vi "E517_Wavegen_Example.vi"(0 "System no.":i32=1 min=1 step=1, 1 "# Wavegenerators":i32, 2 "Programmatic events":T1(array[ring]), 5 "error in":errorcluster, 6 "Enabled":bool[](array[boolean])=[FALSE, FALSE, FALSE, FALSE, FALSE, FALSE, FALSE, FALSE], 7 "# WG cycles":i32[](array[numeric]) format="%#.0f", 9 "SIN_P parameters":cluster{"C":dbl, "A":dbl, "O":dbl}={"C"=500.0, "A"=5.0, "O"=0.0} {"O" format="%.6f"; "A" format="%.6f"; "C" format="%.6f"}, 11 "Firing Wavepoints":i32[][](array[numeric])=[[100, 550], [200, 450], [300, 350]] format="%#.0f", 13 "Append?":bool) -> (16 "Triggerpoints":dbl[][](graph), 17 "Wavetable data":dbl[][](graph), 18 "Recordtable data":dbl[][](graph), 19 "Error out":errorcluster)   [LabVIEW 2011]
doc: "This VI demonstrates how to configure the wave generator, set wave tables, read data recorder tables and set trigger points. The diagram shows how to combine the driver VIs for these tasks. \nThe controls connected to the connector pane exemplify the application. You can modify the connector pane and add controls to meet your requirements. The E517_Wavegen_Example_Caller.vi shows how to call this VI programmatically as a SubVI.\n\nRun E517_Configuration_Setup.vi prior to running this VI.\n\nOn the [Settings] tab you can link wave tables to wave generators if this feature is supported by your controller, adjust wave table and record table rates and configure the wave generator. The current wave generator mode setting (WGO), the actual positions and the servo states are updated continuously.\n \nSelect the desired wave table on the [Wavetables] tab to write a waveform into it or to clean a previously stored waveform. #points in WT shows the actual length of the tables. You can apply controller generated sine waves or host PC generated point-by-point ramp waveforms covering the motion range of the appropriate connected stage. Please consult the Context Help window of the WAV.vi the User Manual of your controller for details on waveform settings. After writing a waveform to the controller all waveforms are read back and displayed automatically. You can read out the wave tables manually, too.\n\nAll further tabs are disabled until you have defined one wave table at least.\n \nConfigure the data recorder on the [Recordtables] tab prior to reading out any data. Each data recorder table must be configured separately by choosing a linked axis and an axis related record option. The contents of the data recorder tables are not read out automatically. Reasonable data is only available if at least one wave generator run has been started since the last power-on / reboot of the controller.\n \nOn the [Triggerpoints] tab you can link axes to triggerlines if this feature is supported by your controller. If you want to output trigger pulses synchronized with the wave generator output, activate the Generator Trigger mode by pressing the Set TWS trigger mode button. The trigger related controls will then be activated. In the matrix you can define the active trigger points for each triggerline. They will be written to the controller's RAM by Set these trigger points. To reset trigger points use Clear all trigger points. In the graphics pane the active trigger points are displayed as bars."
panel:
  out "Number of Triggerlines":i32
  out "SubVI":bool
  out "Running?":bool[](array[boolean])
  in  "Tab Control":T2(tab)
  out "Axes":string[](array[string])
  in  "Recordtable rate":i32=1
  in  "Wavegen":i32[](array[numeric])=[1, 2, 3] format="%#.0f"
  out "# Recordtables":i32
  out "# Wavetables":i32
  out "# Wavegenerators":i32
  out "Servo":bool[](array[boolean])
  in  "Wavetable rate":i32[](array[numeric]) format="%#.0f"
  out "Positions":dbl[](array[numeric])
  out "WGO mode":i32[](array[numeric]) format="%#.0f"
  in  "Start at\nEndpoint":bool[](array[boolean])=[FALSE, FALSE, FALSE, FALSE, FALSE, FALSE, FALSE, FALSE]
  in  "DDL init":bool[](array[boolean])=[FALSE, FALSE, FALSE, FALSE, FALSE, FALSE, FALSE, FALSE]
  in  "DDL enable":bool[](array[boolean])=[FALSE, FALSE, FALSE, FALSE, FALSE, FALSE, FALSE, FALSE]
  in  "Segm.Length":i32=1000
  in  "GWD?":bool
  out "# points in WT":i32[](array[numeric]) format="%#.0f"
  in  "WCL":bool
  out "PNT parameters (indicator)":cluster{"Ao..An-1":dbl[]}
  in  "Write sine":bool
  in  "Add?":bool
  in  "Xo":i32=1
  in  "N":i32=1000
  in  "Write points":bool
  out "Assigned\nwavegenerator":i32
  in  "Wavetable":u16(ring) items=["1", "2", "3"]
  in  "DRC?":bool
  out "Record option":string[](array[string])
  out "Source ID":string[](array[string])
  in  "DRC":bool
  in  "Record option":u16(ring)=1 items=["Target position of axis "=1, "Current position of axis "=2, "Position error of axis "=3, "Voltage of piezo channel "=7, "Control output of axis "=15]
  in  "Axis":u16(ring) items=["A", "B", "C"]
  in  "Record table":u16(ring) items=["1", "2", "3"]
  in  "N:":i32=1000
  in  "X0:":i32=1
  in  "DRR?":bool
  in  "CTO":bool
  in  "TWC":bool
  in  "TWS":bool
  in  "TWS?":bool
  in  "Axis":u16[](array[ring]) items=["A", "B", "C"]
  in  "Clear error":bool
  in  "Stop":bool
  # "E-517 wave generator, data recorder and trigger setting sample program"
  # "This VI demonstrates how to configure the wave generator, set wavetables, read recordtables and set triggerpoints.\nYou can apply controller generated sine waves or host PC generated point-by-point ramp waveforms.\nRun E517_Configuration_Setup.vi prior to running this VI."
  # "Wavegenerator state:"
  # "Wavetable"
  # "1"
  # "2"
  # "3"
  # "4"
  # "5"
  # "6"
  # "7"
  # "8"
  # "Wavegen"
  # "1"
  # "2"
  # "3"
  # "4"
  # "5"
  # "6"
  # "7"
  # "8"
  # "1"
  # "2"
  # "3"
  # "4"
  # "5"
  # "6"
  # "7"
  # "8"
  # "1black 2red 3green 4cyan 5yelllow 6purple 7orange 8blue"
  # "1"
  # "2"
  # "3"
  # "4"
  # "5"
  # "6"
  # "7"
  # "8"
  # "1black 2red 3green 4cyan 5yelllow 6purple 7orange 8blue"
  # "Trigger"
  # "1"
  # "2"
  # "3"
  # "4"
  # "5"
  # "6"
  # "1black 2red 3green 4blue 5yelllow 6purple"
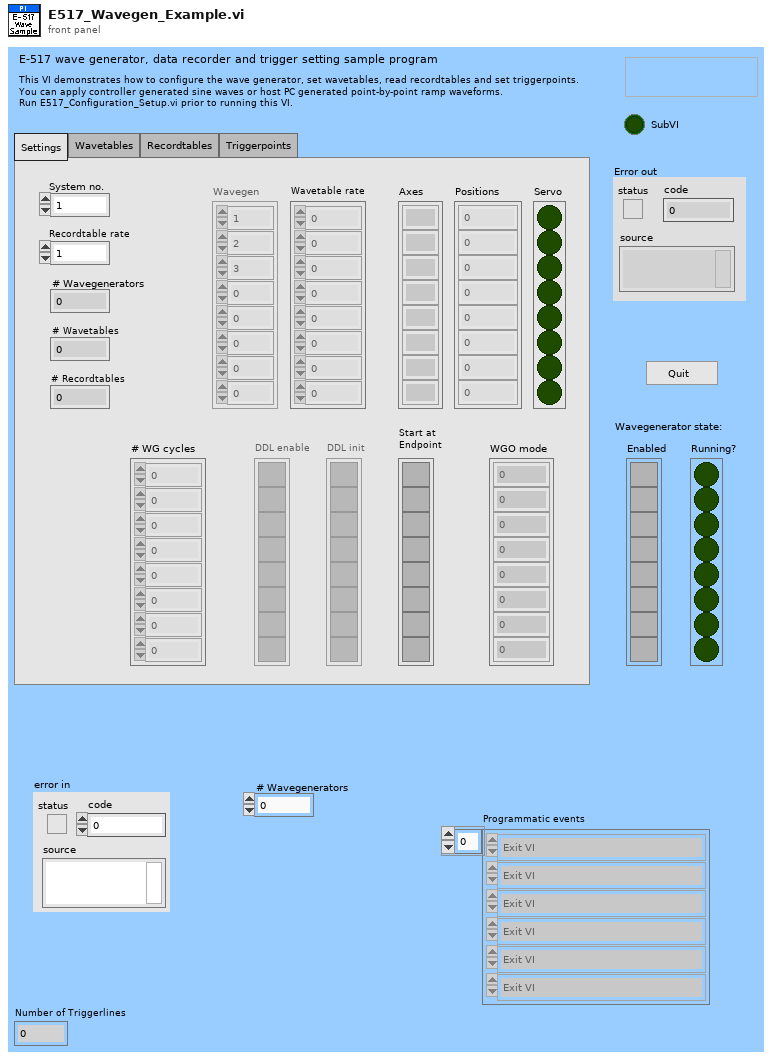
[diagram p1: front panel]
types:
  T1 = enum16{"Exit VI", "Set trigger mode", "Set recordtable rate", "Set wavetable rate", "Write sine", "Read wavetable", "Read recordtable", "Enable/disable wavegen", "Set number of wavegen cycles", "Clear wavetable", "Configure data recorder", "Assign wavetable to wavegen", "Read trigger points", "Set trigger points", "Clear trigger points", "Assign axes to triggerlines", "Write ramp waveform", "Set DDL enable", "Set DDL init", "Set Start at endpoint"}[]
  T2 = enum32{"Settings", "Wavetables", "Recordtables", "Triggerpoints"}
  T3 = enum32{"Page Enabled", "Page Disabled", "Page Disabled & Grayed"}
  T4 = enum16{"Position Distance", "Position Distance & Wait Time", "OnTarget", "MinMax Threshold", "Generator Trigger (TWS)", "Motion Error", "In Motion"}
  T5 = enum16{"Unused", "TriggerStep", "Axis", "TriggerMode", "TriggerDelay", "MinThreshold", "MaxThreshold", "Polarity", "StartThreshold", "StopThreshold"}
  T6 = enum16{"Position Distance", "Position Distance & Wait Time", "OnTarget", "MinMax Threshold", "Generator Trigger (TWS)", "Motion Error", "In Motion"}[]
  T7 = enum16{"Unused", "TriggerStep", "Axis", "TriggerMode", "TriggerDelay", "MinThreshold", "MaxThreshold", "Polarity", "StartThreshold", "StopThreshold"}[]
  T8 = enum16{"Exit VI", "Set trigger mode", "Set recordtable rate", "Set wavetable rate", "Write sine", "Read wavetable", "Read recordtable", "Enable/disable wavegen", "Set number of wavegen cycles", "Clear wavetable", "Configure data recorder", "Assign wavetable to wavegen", "Read trigger points", "Set trigger points", "Clear trigger points", "Assign axes to triggerlines", "Write ramp waveform", "Set DDL enable", "Set DDL init", "Set Start at endpoint"}
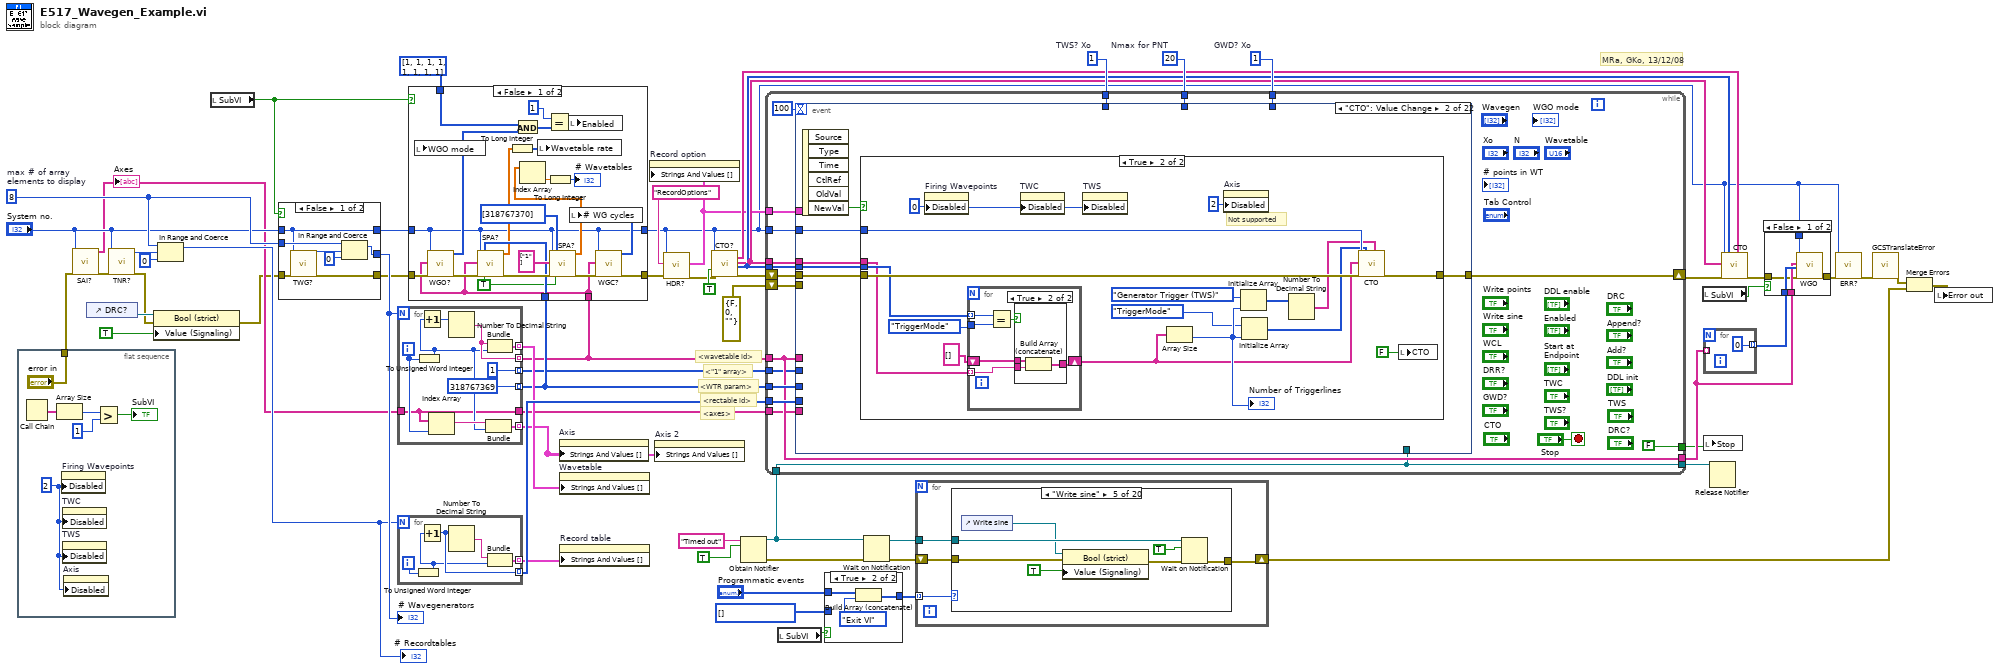
[diagram p0: block diagram]
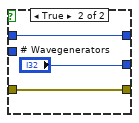
[diagram p3: hidden frame]
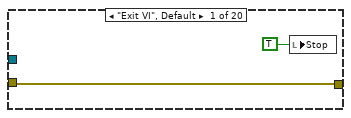
[diagram p6: hidden frame]
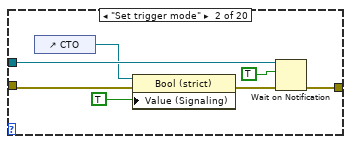
[diagram p7: hidden frame]
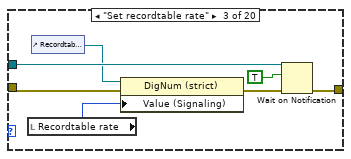
[diagram p8: hidden frame]
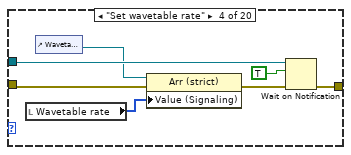
[diagram p9: hidden frame]
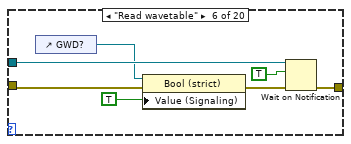
[diagram p10: hidden frame]
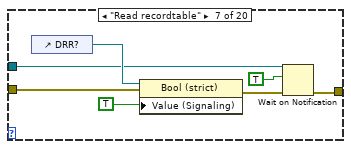
[diagram p11: hidden frame]
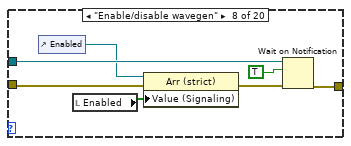
[diagram p12: hidden frame]
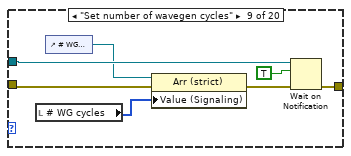
[diagram p13: hidden frame]
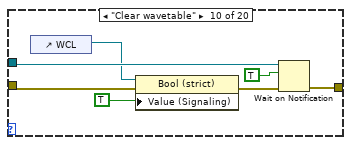
[diagram p14: hidden frame]
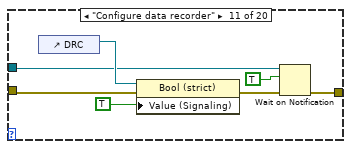
[diagram p15: hidden frame]
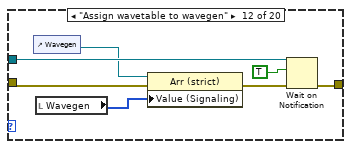
[diagram p16: hidden frame]
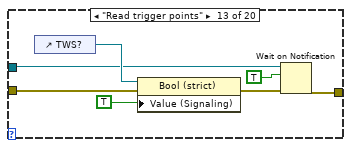
[diagram p17: hidden frame]
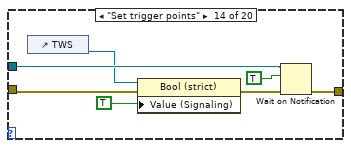
[diagram p18: hidden frame]
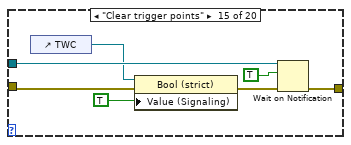
[diagram p19: hidden frame]
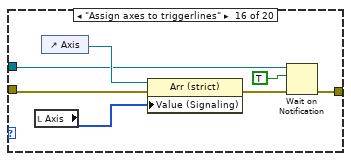
[diagram p20: hidden frame]
diagram:
  w14 = T1 [] items=["Exit VI", "Set trigger mode", "Set recordtable rate", "Set wavetable rate", "Write sine", "Read wavetable", "Read recordtable", "Enable/disable wavegen", "Set number of wavegen cycles", "Clear wavetable", "Configure data recorder", "Assign wavetable to wavegen", "Read trigger points", "Set trigger points", "Clear trigger points", "Assign axes to triggerlines", "Write ramp waveform", "Set DDL enable", "Set DDL init", "Set Start at endpoint"] ("Programmatic events")
  w48 = 20  # Nmax for PNT
  w49 = 1  # TWS? Xo
  w50 = 1  # GWD? Xo
  w9 = 8  # max # of array  elements to display
  # "<axes>"
  # "MRa, GKo, 13/12/08"
  # "<wavetable id>"
  # "<rectable id>"
  # "<\"1\" array>"
  # "<WTR param>"
  n1 = flat-sequence {
    tunnel: ["error in"] -> w18
    frame #0 {
      w62 = u8 2 ("Disabled")
      n2 = Call Chain() -> (call chain=w67:string[])
      n3 = Array Size(array=w67) -> (size(s)=w66:i32)
      n4 = property on="Firing Wavepoints" class="Arr (strict)"("Disabled"=w62) -> ()  [unwired: 2 in, 2 out]
      n5 = property on="TWC" class="Bool (strict)"("Disabled"=w62) -> ()  [unwired: 2 in, 2 out]
      n6 = property on="TWS" class="Bool (strict)"("Disabled"=w62) -> ()  [unwired: 2 in, 2 out]
      n7 = property on="Axis" class="Arr (strict)"("Disabled"=w62) -> ()  [unwired: 2 in, 2 out]
      n8 = Greater?(x=w66, y=1) -> (0:→"SubVI":bool)
    }
  }
  n9 = call "SAI?.vi"("System no."="System no.", "error in"=w18) -> ("Conn. axes"=w4:string[], "error out"=w52:errorcluster)  [unwired: 3 in, 13 out]
  "Axes" <- w4
  n10 = control-ref of="DRC?"() -> (w46:refnum<vi>)
  n11 = call "TNR?.vi"("System no."="System no.", "error in"=w52) -> ("Number of Rec. tables"=w57:i32, "error out"=w13:errorcluster)  [unwired: 16 out]
  n12 = property class="Bool (strict)"(reference=w46, error in=w13, "Value (Signaling)"=TRUE ("TWC")) -> (error out=w2:errorcluster)  [unwired: 1 out]
  n13 = In Range and Coerce(upper limit=w9, x=w57, lower limit=0) -> (coerced(x)=w6:i32)  [unwired: 1 out]
  "# Recordtables" <- w6
  n14 = local read "SubVI"() -> (w11:bool)
  n15 = case shown="False" w11 {
    tunnel: [w74 w76] -> w10
    tunnel: w2 -> [w73 w76]
    tunnel: w9 -> [w71 _]
    tunnel: [w69 "# Wavegenerators"] -> w12
    tunnel: "System no." -> [w68 w77]
    tunnel: [w68 w77] -> w7
    frame False {
      n16 = call "TWG?.vi"("System no."=w68, "error in"=w73) -> ("Number of wave generators"=w72:i32, "error out"=w74:errorcluster)  [unwired: 16 out]
      n17 = In Range and Coerce(upper limit=w71, x=w72, lower limit=0) -> (coerced(x)=w69:i32)  [unwired: 1 out]
    }
    frame True {
    }
  }
  "# Wavegenerators" <- w12
  n18 = for {
    N: w12 -> [_]
    tunnel: [w86] -> w59 mode=indexing
    tunnel: [w81] -> w17 mode=indexing
    tunnel: [318767369 ("Numeric")] -> w56 mode=indexing
    tunnel: [1 ("Number of wave generators")] -> w51 mode=indexing
    tunnel: w4 -> [w78]
    tunnel: [w80] -> w1 mode=indexing
    tunnel: [w78] -> w3
    i -> [w83]
    n19 = To Unsigned Word Integer(number=w83) -> (unsigned 16bit integer=w79:u16)
    n20 = Increment(x=w79) -> (x+1=w87:u16)
    n21 = Index Array(array=w78, index=w83) -> (element=w82:string)
    n22 = Number To Decimal String(number=w87) -> (decimal integer string=w81:string)  [unwired: 1 out]
    n23 = Bundle("String"=w82, w79) -> (w80:cluster{"String":string, u16})  [unwired: 1 out]
    n24 = Bundle(w81, w79) -> (w86:cluster{string, u16})  [unwired: 1 out]
  }
  n25 = for {
    N: w6 -> [_]
    tunnel: [w92] -> w60 mode=indexing
    tunnel: [w90] -> w61 mode=indexing
    i -> [w89]
    n26 = To Unsigned Word Integer(number=w89) -> (unsigned 16bit integer=w88:u16)
    n27 = Increment(x=w88) -> (x+1=w90:u16)
    n28 = Number To Decimal String(number=w90) -> (decimal integer string=w91:string)  [unwired: 1 out]
    n29 = Bundle(w91, w88) -> (w92:cluster{string, u16})  [unwired: 1 out]
  }
  n30 = case shown="False" w11 {
    tunnel: w10 -> [w114 w115]
    tunnel: w56 -> [w109 _]
    tunnel: [w108 w115] -> w24
    tunnel: w7 -> [w94 w116]
    tunnel: i32[] [1, 1, 1, 1, 1, 1, 1, 1] ("WGO parameter") -> [w104 _]
    tunnel: [w94 w116] -> w19
    tunnel: w17 -> [w93 _]
    frame False {
      w97 = TRUE ("Parameter no. format \n(Decimal: FALSE)")
      n31 = call "WGO?.vi"("System no."=w94, "Axes to query"=w93, "error in"=w114) -> ("WGO parameter"=w103:i32[], "error out"=w111:errorcluster)  [unwired: 2 in, 13 out]
      n32 = local write "WGO mode"(w103) -> ()
      n33 = call "SPA?.vi"("System no."=w94, "Axes to query"=w93, "error in"=w111, "Parameter no. (hex)"=w109, "Parameter no. format \n(Decimal: FALSE)"=w97) -> ("Parameter value"=w101:dbl[], "error out"=w110:errorcluster)  [unwired: 2 in, 11 out]
      n34 = To Long Integer(number=w101) -> (32bit integer=w102:i32[])
      n35 = And(x=w104, y=w103) -> (x .and. y?=w105:i32[])
      n36 = local write "Wavetable rate"(w102) -> ()
      n37 = Equal?(x=1, y=w105) -> (x = y?=w107:bool[])
      n38 = call "SPA?.vi"("System no."=w94, "Axes to query"=string[] ["1"], "error in"=w110, "Parameter no. (hex)"=u32[] [318767370], "Parameter no. format \n(Decimal: FALSE)"=w97) -> ("Parameter value"=w95:dbl[], "error out"=w113:errorcluster)  [unwired: 2 in, 11 out]
      n39 = Index Array(array=w95) -> (element=w100:dbl)  [unwired: 1 in]
      n40 = To Long Integer(number=w100) -> (32bit integer=→"# Wavetables":i32)
      n41 = local write "Enabled"(w107) -> ()
      n42 = call "WGC?.vi"("System no."=w94, "Axes to query"=w93, "error in"=w113) -> ("Cycles"=w98:i32[], "error out"=w108:errorcluster)  [unwired: 2 in, 13 out]
      n43 = local write "# WG cycles"(w98) -> ()
    }
    frame True {
    }
  }
  n44 = property on="Axis" class="Ring (strict)"("Strings And Values []"=w1) -> ()  [unwired: 2 in, 2 out]
  n45 = property on="Wavetable" class="Ring (strict)"("Strings And Values []"=w59) -> ()  [unwired: 2 in, 2 out]
  n46 = property on="Record table" class="Ring (strict)"("Strings And Values []"=w60) -> ()  [unwired: 2 in, 2 out]
  n47 = property on="Axis 2" class="Ring (strict)"("Strings And Values []"=w1) -> ()  [unwired: 2 in, 2 out]
  n48 = call "HDR?.vi"("System no."=w19, "Section header"="RecordOptions" ("Header"), "error in"=w24) -> ("Enum values"=w21:cluster{"token string":string, i32}[], "error out"=w23:errorcluster)  [unwired: 15 out]
  n49 = property on="Record option" class="Ring (strict)"("Strings And Values []"=w21) -> ()  [unwired: 2 in, 2 out]
  n50 = call "CTO?.vi"("System no."=w19, "All Triggers?"=TRUE, "error in"=w23) -> ("Parameter value"=w39:string[], "TriggerOut to query out"=w37:string[], "CTO parameter ID out"=w38:i32[], "error out"=w45:errorcluster)  [unwired: 2 in, 11 out]
  n51 = Obtain Notifier(name (unnamed)="Timed out", notification data type=TRUE ("GWD?")) -> (notifier out=w28:refnum<notifier>, error out=w31:errorcluster)  [unwired: 2 in, 1 out]
  n52 = while {
    tunnel: w19 -> [w126]
    shift-right: [w130] -> w41
    shift-left: w45 -> [w134]
    tunnel: w17 -> [w128]
    tunnel: w61 -> [w132]
    tunnel: w21 -> [w131]
    tunnel: w56 -> [w129]
    tunnel: [w128] -> w42
    shift-left: errorcluster {"status"=FALSE, "code"=0, "source"=""} ("error in") -> [w127]
    tunnel: w51 -> [w125]
    tunnel: w50 -> [w124]
    tunnel: w49 -> [w123]
    tunnel: w48 -> [w122]
    tunnel: w38 -> [w121]
    tunnel: w37 -> [w120]
    tunnel: [FALSE ("Stop")] -> w35
    tunnel: [w118] -> w32
    tunnel: w28 -> [w118]
    tunnel: w3 -> [w117]
    stop <- "Stop" stop-if-true
    n53 = event shown="[1] \"CTO\": Value Change" {
      selector: _ -> [_ _ _ _ _ _ _ _ _ _ _ _ _ _ _ _ _ _ _ _ _ _]
      dyn-events: _ -> [_ _ _ _ _ _ _ _ _ _ _ _ _ _ _ _ _ _ _ _ _ _]
      timeout: 100 -> [_ _ _ _ _ _ _ _ _ _ _ _ _ _ _ _ _ _ _ _ _ _]
      tunnel: w134 -> [w143 w190 w222 w230 w233 w263 w268 w304 w333 w338 w341 w365 w389 w415 w419 w443 w471 w485 w506 w548 w557 w566]
      tunnel: w126 -> [w147 w188 w220 w226 w232 _ w267 w303 w324 w337 w340 w364 w388 _ w418 w442 w469 w488 w505 _ _ _]
      tunnel: w128 -> [_ _ _ w225 w234 _ w269 w305 w323 w336 w342 _ w390 _ _ _ _ _ w504 _ _ _]
      tunnel: w132 -> [_ _ _ _ _ _ _ w302 _ _ _ w363 _ _ _ _ _ _ _ _ _ _]
      tunnel: w131 -> [_ _ _ _ _ _ _ _ _ _ _ w362 w387 _ _ _ _ _ _ _ _ _]
      tunnel: [w144 w189 w221 w229 w231 w263 w266 w301 w325 w334 w339 w361 w386 w415 w417 w441 w470 w486 w502 w548 w557 w566] -> w130
      tunnel: w129 -> [_ _ _ w224 _ _ _ _ _ _ _ _ _ _ _ _ _ _ _ _ _ _]
      tunnel: w127 -> [w142 _ _ _ _ _ _ _ _ _ _ _ _ _ _ _ _ _ _ _ _ _]
      tunnel: w125 -> [_ _ _ _ _ _ w265 _ _ _ _ _ _ _ _ _ _ _ _ _ _ _]
      tunnel: w124 -> [_ _ _ _ _ _ w264 _ _ _ _ _ _ _ _ _ _ _ _ _ _ _]
      tunnel: w123 -> [_ _ _ _ _ _ _ _ _ _ _ _ _ _ w416 _ _ _ _ _ _ _]
      tunnel: w122 -> [_ _ _ _ _ _ _ _ _ _ _ _ _ _ _ _ _ _ w501 _ _ _]
      tunnel: w121 -> [_ w187 _ _ _ _ _ _ _ _ _ _ _ _ _ _ _ _ _ _ _ _]
      tunnel: w120 -> [_ w186 _ _ _ _ _ _ _ _ _ _ _ _ _ _ _ _ _ _ _ _]
      tunnel: w118 -> [w136 _ _ _ _ _ _ _ _ _ _ _ _ _ _ _ _ _ _ _ _ _]
      tunnel: w117 -> [_ _ _ _ _ _ _ _ _ _ _ w360 _ _ _ _ _ w492 _ _ _ _]
      event Timeout {
        n54 = event-data() -> ()  [unwired: 3 out]
        n55 = Unbundle By Name(w142) -> ("status"=w140:bool)
        n56 = call "ERR?.vi"("System no."=w147, "error in"=w143) -> ("error out"=w138:errorcluster)  [unwired: 17 out]
        n57 = Unbundle By Name(w138) -> ("status"=w141:bool)
        n58 = Not Equal?(x=w141, y=w140) -> (x != y?=w139:bool)
        n59 = case shown="False" w139 {
          tunnel: w138 -> [w148 w150]
          tunnel: [w148 w149] -> w146
          frame False {
          }
          frame True {
            n60 = call "GCSTranslateError.vi"("error in"=w150) -> ("error out"=w149:errorcluster)  [unwired: 18 out]
          }
        }
        n61 = case shown="No Error" w146 {
          selector: w146 -> [w151 w181]
          tunnel: [w152 w182] -> w144
          tunnel: w147 -> [w164 _]
          frame No Error {
            w154 = TRUE  # All axes?
            n62 = local read "# points in WT"() -> (w158:i32[])
            n63 = Greater Than 0?(x=w158) -> (x > 0?=w157:bool[])
            n64 = Or Array Elements(Boolean array=w157) -> (logical OR=w159:bool)
            n65 = call "#9.vi"("System no."=w164, "error in"=w151) -> ("WG running?"=→"Running?":bool[], "error out"=w167:errorcluster)  [unwired: 16 out]
            n66 = Select(t=T3."Page Enabled" ("Page Enabled State"), s=w159, f=T3."Page Disabled & Grayed" ("Page Enabled State")) -> (s? t:f=w162:T3)
            n67 = call "POS?.vi"("System no."=w164, "All axes?"=w154, "error in"=w167) -> ("Position"=→"Positions":dbl[], "error out"=w165:errorcluster)  [unwired: 2 in, 13 out]
            n68 = call "SVO?.vi"("System no."=w164, "All axes?"=w154, "error in"=w165) -> ("Servo status?"=→"Servo":bool[], "error out"=w153:errorcluster)  [unwired: 2 in, 13 out]
            n69 = property on="Tab Control" class="TabCtl (strict)"(error in=w153) -> (error out=w156:errorcluster, "Pages"=w155:refnum<vi>[])  [unwired: 1 in, 1 out]
            n70 = for {
              shift-right: [w174] -> w152
              shift-left: w156 -> [w175]
              tunnel: w155 -> [w173] mode=indexing
              tunnel: w162 -> [w172]
              i -> [w171]
              n71 = Greater?(x=w171, y=1) -> (0:w169:bool)
              n72 = case shown="True" w169 {
                tunnel: w175 -> [w176 w180]
                tunnel: [w176 w179] -> w174
                tunnel: w173 -> [_ w178]
                tunnel: w172 -> [_ w177]
                frame False {
                }
                frame True {
                  n73 = property class="Page"(reference=w178, error in=w180, "Page Enabled State"=w177) -> (error out=w179:errorcluster)  [unwired: 1 out]
                }
              }
            }
          }
          frame Error {
            n74 = Select(t=errorcluster {"status"=FALSE, "code"=0, "source"=""}, s="Clear error", f=w181) -> (s? t:f=w182:errorcluster)
          }
        }
        "Error out" <- w144
        n75 = Unbundle By Name(w144) -> ("status"=w145:bool)
        n76 = property on="Clear error" class="Bool"("Visible"=w145) -> ()  [unwired: 2 in, 2 out]
        n77 = Send Notification(notification=TRUE, notifier=w136) -> ()  [unwired: 1 in, 2 out]
      }
      event "CTO": Value Change {
        n78 = event-data() -> ("NewVal"=w185:bool)  [unwired: 6 out]
        n79 = case shown="True" w185 {
          tunnel: w190 -> [w191 w208]
          tunnel: [w191 w207] -> w189
          tunnel: w188 -> [_ w206]
          tunnel: w187 -> [_ w205]
          tunnel: w186 -> [_ w204]
          frame False {
          }
          frame True {
            w193 = u8 0 ("Disabled")
            # "Not supported"
            n80 = property on="Firing Wavepoints" class="Arr (strict)"("Disabled"=w193) -> ()  [unwired: 2 in, 2 out]
            n81 = for {
              tunnel: w205 -> [w214] mode=indexing
              tunnel: w204 -> [w210] mode=indexing
              shift-right: [w211] -> w196
              shift-left: string[] [] -> [w212]
              tunnel: T5."TriggerMode" -> [w209]
              n82 = Equal?(x=w214, y=w209) -> (x = y?=w213:bool)
              n83 = case shown="True" w213 {
                tunnel: w212 -> [w215 w218]
                tunnel: [w215 w217] -> w211
                tunnel: w210 -> [_ w216]
                frame False {
                }
                frame True {
                  n84 = Build Array (concatenate)(w218, w216) -> (w217:string[])
                }
              }
            }
            n85 = property on="TWC" class="Bool (strict)"("Disabled"=w193) -> ()  [unwired: 2 in, 2 out]
            n86 = property on="TWS" class="Bool (strict)"("Disabled"=w193) -> ()  [unwired: 2 in, 2 out]
            n87 = Array Size(array=w196) -> (size(s)=w202:i32)
            "Number of Triggerlines" <- w202
            n88 = property on="Axis" class="Arr (strict)"("Disabled"=u8 2) -> ()  [unwired: 2 in, 2 out]
            n89 = Initialize Array(T4."Generator Trigger (TWS)", w202) -> (w201:T6)
            n90 = Initialize Array(T5."TriggerMode", w202) -> (w194:T7)
            n91 = Number To Decimal String(number=w201) -> (decimal integer string=w200:string[])  [unwired: 1 out]
            n92 = call "CTO.vi"("System no."=w206, "TriggerOut to set"=w196, "error in"=w208, "CTO parameter ID"=w194, "Parameter value"=w200) -> ("error out"=w207:errorcluster)  [unwired: 1 in, 13 out]
            n93 = local write "CTO"(FALSE ("CTO")) -> ()
          }
        }
      }
      event "Recordtable rate": Value Change {
        n94 = event-data() -> ()  [unwired: 7 out]
        n95 = call "RTR.vi"("System no."=w220, "Table rate"="Recordtable rate", "error in"=w222) -> ("error out"=w221:errorcluster)  [unwired: 16 out]
      }
      event "Wavetable rate": Value Change {
        n96 = event-data() -> ()  [unwired: 7 out]
        n97 = To Double Precision Float(number="Wavetable rate") -> (double precision float=w227:dbl[])
        n98 = call "SPA.vi"("System no."=w226, "Axis to set"=w225, "Parameter value"=w227, "error in"=w230, "Parameter no. format \n(Decimal: FALSE)"=TRUE ("Parameter no. format \n(Decimal: FALSE)"), "Parameter number (hex)"=w224) -> ("error out"=w229:errorcluster)  [unwired: 4 in, 9 out]
      }
      event "Write sine": Value Change {
        n99 = event-data() -> ("NewVal"=w235:bool)  [unwired: 6 out]
        n100 = case shown="True" w235 {
          tunnel: w233 -> [w236 w239]
          tunnel: [w236 w238] -> w231
          tunnel: w232 -> [_ w243]
          tunnel: w234 -> [_ w244]
          frame False {
          }
          frame True {
            w254 = u16 4 items=["SIN", "POL", "TAN", "PNT", "SIN_P", "LIN", "RAMP"] ("Waveform")
            n101 = local read "Wavetable"() -> (w242:u16)
            n102 = local read "N"() -> (w247:i32)
            n103 = local read "Append?"() -> (w251:bool)
            n104 = local read "Xo"() -> (w249:i32)
            n105 = local read "Add?"() -> (w250:bool)
            n106 = Index Array(array=w244, index=w242) -> (element=w253:string)
            n107 = Build Array(w253) -> (w252:string[])
            n108 = call "WAV.vi"("System no."=w243, "Waveform"=w254, "Affected axes"=w252, "Append? (&)"=w251, "Add? (+)"=w250, "error in"=w239, "Xo"=w249, "N"=w247, "Segment length"="Segm.Length", "SIN_P Parameters"="SIN_P parameters") -> ("error out"=w245:errorcluster)  [unwired: 8 in, 9 out]
            n109 = call "Wait for controller ready.vi"("System no."=w243, "error in"=w245) -> ("error out"=w241:errorcluster)  [unwired: 2 in, 15 out]
            n110 = local read "SubVI"() -> (w237:bool)
            n111 = case shown="False" w237 {
              tunnel: w241 -> [w256 w259]
              tunnel: [w255 w259] -> w238
              frame False {
                n112 = control-ref of="GWD?"() -> (w258:refnum<vi>)
                n113 = property class="Bool (strict)"(reference=w258, error in=w256, "Value (Signaling)"=TRUE ("GWD?")) -> (error out=w255:errorcluster)  [unwired: 1 out]
              }
              frame True {
              }
            }
            n114 = local write "Write sine"(FALSE ("Write sine")) -> ()
          }
        }
      }
      event "Wavetable": Value Change {
        n115 = event-data() -> ("NewVal"=w262:u16)  [unwired: 6 out]
        n116 = local read "Wavegen"() -> (w261:i32[])
        n117 = Index Array(array=w261, index=w262) -> (element=→"Assigned\nwavegenerator":i32)
      }
      event "GWD?": Value Change {
        n118 = event-data() -> ("NewVal"=w270:bool)  [unwired: 6 out]
        n119 = case shown="True" w270 {
          tunnel: w268 -> [w271 w281]
          tunnel: [w271 w272] -> w266
          tunnel: w267 -> [_ w278]
          tunnel: w269 -> [_ w277]
          tunnel: w265 -> [_ w276]
          tunnel: w264 -> [_ w275]
          frame False {
          }
          frame True {
            n120 = call "WAV?.vi"("System no."=w278, "Axes to query"=w277, "Parameter no."=w276, "error in"=w281) -> ("WAV Parameter value"=w279:dbl[], "error out"=w274:errorcluster)  [unwired: 14 out]
            n121 = To Long Integer(number=w279) -> (32bit integer=w280:i32[])
            n122 = local write "# points in WT"(w280) -> ()
            n123 = for {
              tunnel: w278 -> [w288]
              tunnel: w277 -> [w287] mode=indexing
              tunnel: [w286] -> w282 mode=indexing
              shift-right: [w289] -> w272
              shift-left: w274 -> [w290]
              tunnel: w280 -> [w284] mode=indexing
              tunnel: w275 -> [w283]
              n124 = Greater Than 0?(x=w284) -> (x > 0?=w285:bool)
              n125 = case shown="True" w285 {
                tunnel: w290 -> [w292 w299]
                tunnel: [w292 w298] -> w289
                tunnel: w288 -> [_ w297]
                tunnel: w287 -> [_ w296]
                tunnel: [dbl[] [] ("Waveform points") w295] -> w286
                tunnel: w284 -> [_ w294]
                tunnel: w283 -> [_ w293]
                frame False {
                }
                frame True {
                  n126 = call "GWD?.vi"("System no."=w297, "Query axis"=w296, "error in"=w299, "Xo"=w293, "N"=w294) -> ("Waveform points"=w295:dbl[], "error out"=w298:errorcluster)  [unwired: 6 in, 7 out]
                }
              }
            }
            "Wavetable data" <- w282
            n127 = local write "GWD?"(FALSE ("GWD?")) -> ()
          }
        }
      }
      event "DRR?": Value Change {
        n128 = event-data() -> ("NewVal"=w300:bool)  [unwired: 6 out]
        n129 = case shown="True" w300 {
          tunnel: w304 -> [w306 w310]
          tunnel: [w306 w316] -> w301
          tunnel: w303 -> [_ w308]
          tunnel: w305 -> [_ _]
          tunnel: w302 -> [_ w311]
          frame False {
          }
          frame True {
            n130 = call "WGR.vi"("System no."=w308, "error in"=w310) -> ("error out"=w309:errorcluster)  [unwired: 17 out]
            n131 = call "DRR?.vi"("System no."=w308, "Rec. table IDs"=w311, "error in"=w309, "Xo"="X0:", "N"="N:") -> ("Data"=w313:dbl[][], "error out"=w316:errorcluster)  [unwired: 2 in, 11 out]
            n132 = Transpose 2D Array(2D array=w313) -> (transposed array=→"Recordtable data":dbl[][])
            n133 = local write "DRR?"(FALSE ("DRR?")) -> ()
          }
        }
      }
      event "Enabled": Value Change {
        w329 = 1
        n134 = event-data() -> ("NewVal"=w327:bool[])  [unwired: 6 out]
        n135 = Array Size(array=w323) -> (size(s)=w322:i32)
        n136 = local read "WGO mode"() -> (w318:i32[])
        n137 = Initialize Array(1, w322) -> (w319:i32[])
        n138 = Boolean To (0,1)(Boolean=w327) -> (0, 1=w328:i16[])
        n139 = local read "SubVI"() -> (w317:bool)
        n140 = Multiply(x=w328, y=w329) -> (x*y=w331:i32[])
        n141 = Not(x=w329) -> (.not. x?=w330:i32)
        n142 = Select(t=w319, s=w317, f=w318) -> (s? t:f=w320:i32[])
        n143 = And(x=w320, y=w330) -> (x .and. y?=w332:i32[])
        n144 = Or(x=w332, y=w331) -> (x .or. y?=w326:i32[])
        n145 = call "WGO.vi"("System no."=w324, "Affected axes"=w323, "WGO Parameter"=w326, "error in"=w333) -> ("error out"=w325:errorcluster)  [unwired: 6 in, 9 out]
        n146 = local write "WGO mode"(w326) -> ()
      }
      event "# WG cycles": Value Change {
        n147 = event-data() -> ()  [unwired: 7 out]
        n148 = call "WGC.vi"("System no."=w337, "Affected axes"=w336, "Cycles"="# WG cycles", "error in"=w338) -> ("error out"=w334:errorcluster)  [unwired: 15 out]
      }
      event "WCL": Value Change {
        n149 = event-data() -> ("NewVal"=w343:bool)  [unwired: 6 out]
        n150 = case shown="True" w343 {
          tunnel: w341 -> [w344 w354]
          tunnel: [w344 w348] -> w339
          tunnel: w340 -> [_ w353]
          tunnel: w342 -> [_ w352]
          frame False {
          }
          frame True {
            n151 = local read "Wavetable"() -> (w347:u16)
            n152 = Index Array(array=w352, index=w347) -> (element=w351:string)
            n153 = Build Array(w351) -> (w350:string[])
            n154 = call "WCL.vi"("System no."=w353, "WCL axes"=w350, "error in"=w354) -> ("error out"=w349:errorcluster)  [unwired: 6 in, 10 out]
            n155 = local read "SubVI"() -> (w346:bool)
            n156 = case shown="False" w346 {
              tunnel: w349 -> [w356 w359]
              tunnel: [w355 w359] -> w348
              frame False {
                n157 = control-ref of="GWD?"() -> (w358:refnum<vi>)
                n158 = property class="Bool (strict)"(reference=w358, error in=w356, "Value (Signaling)"=TRUE ("GWD?")) -> (error out=w355:errorcluster)  [unwired: 1 out]
              }
              frame True {
              }
            }
            n159 = local write "WCL"(FALSE ("WCL")) -> ()
          }
        }
      }
      event "DRC": Value Change {
        n160 = event-data() -> ("NewVal"=w366:bool)  [unwired: 6 out]
        n161 = case shown="True" w366 {
          tunnel: w365 -> [w367 w380]
          tunnel: [w367 w371] -> w361
          tunnel: w364 -> [_ w377]
          tunnel: w360 -> [_ w379]
          tunnel: w363 -> [_ w376]
          tunnel: w362 -> [_ _]
          frame False {
          }
          frame True {
            # "It's always connected\nwavegen 1 <-> axis 1,\n2 <-> 2, 3 <-> 3, etc."
            n162 = Index Array(array=w379, index="Axis") -> (element=w368:string)
            n163 = Index Array(array=w376, index="Record table") -> (element=w378:u16)
            n164 = call "DRC.vi"("System no."=w377, "Rec. table"=w378, "Rec. option"="Record option", "error in"=w380, "Source ID"=w368) -> ("error out"=w372:errorcluster)  [unwired: 1 in, 13 out]
            n165 = local read "SubVI"() -> (w370:bool)
            n166 = case shown="False" w370 {
              tunnel: w372 -> [w382 w385]
              tunnel: [w381 w385] -> w371
              frame False {
                n167 = control-ref of="DRC?"() -> (w384:refnum<vi>)
                n168 = property class="Bool (strict)"(reference=w384, error in=w382, "Value (Signaling)"=TRUE ("TWC")) -> (error out=w381:errorcluster)  [unwired: 1 out]
              }
              frame True {
              }
            }
            n169 = local write "DRC"(FALSE ("DRC")) -> ()
          }
        }
      }
      event "DRC?": Value Change {
        n170 = event-data() -> ("NewVal"=w391:bool)  [unwired: 6 out]
        n171 = case shown="True" w391 {
          tunnel: w389 -> [w392 w397]
          tunnel: [w392 w394] -> w386
          tunnel: w388 -> [_ w400]
          tunnel: w390 -> [_ _]
          tunnel: w387 -> [_ w398]
          frame False {
          }
          frame True {
            n172 = call "DRC?.vi"("System no."=w400, "error in"=w397) -> ("Rec. option"=w399:i32[], "Source ID"=→"Source ID":string[], "error out"=w394:errorcluster)  [unwired: 2 in, 13 out]
            n173 = for {
              tunnel: w399 -> [w405] mode=indexing
              tunnel: [w404] -> w396 mode=indexing
              tunnel: w398 -> [w401]
              n174 = Array Size(array=w401) -> (size(s)=w403:i32)
              n175 = Decrement(x=w403) -> (x-1=w402:i32)
              n176 = while {
                tunnel: w401 -> [w414] mode=indexing
                tunnel: [w412] -> w404
                tunnel: w405 -> [w411]
                tunnel: w402 -> [w409]
                i -> [w410]
                stop <- w408 stop-if-true
                n177 = Unbundle(w414) -> ("token string"=w412:string, w413:i32)
                n178 = Greater Or Equal?(x=w410, y=w409) -> (x >= y?=w407:bool)
                n179 = Equal?(x=w413, y=w411) -> (x = y?=w406:bool)
                n180 = Or(x=w406, y=w407) -> (x .or. y?=w408:bool)
              }
            }
            "Record option" <- w396
            n181 = local write "DRC?"(FALSE ("DRC?")) -> ()
          }
        }
      }
      event "Wavegen": Value Change {
        # "Not supported by this controller"
        n182 = event-data() -> ()  [unwired: 7 out]
      }
      event "TWS?": Value Change {
        n183 = event-data() -> ("NewVal"=w420:bool)  [unwired: 6 out]
        n184 = case shown="True" w420 {
          tunnel: w419 -> [w421 w433]
          tunnel: [w421 w426] -> w417
          tunnel: w418 -> [_ w432]
          tunnel: w416 -> [_ w424]
          frame False {
          }
          frame True {
            n185 = local read "Number of Triggerlines"() -> (w422:i32)
            n186 = local read "# points in WT"() -> (w431:i32[])
            n187 = for {
              tunnel: w431 -> [w436] mode=indexing
              shift-right: [w438] -> w425
              shift-left: 0 -> [w437]
              n188 = Greater?(x=w436, y=w437) -> (0:w439:bool)
              n189 = Select(t=w436, s=w439, f=w437) -> (s? t:f=w438:i32)
            }
            n190 = for {
              N: w422 -> [_]
              tunnel: [w434] -> w429 mode=indexing
              i -> [w435]
              n191 = Increment(x=w435) -> (x+1=w434:i32)
            }
            n192 = call "TWS?.vi"("System no."=w432, "TriggerOut to query"=w429, "error in"=w433, "Xo"=w424, "N"=w425, "Nmax"=w425) -> ("Data"=w428:dbl[][], "error out"=w426:errorcluster)  [unwired: 1 in, 11 out]
            n193 = Transpose 2D Array(2D array=w428) -> (transposed array=→"Triggerpoints":dbl[][])
            n194 = local write "TWS?"(FALSE ("TWS?")) -> ()
          }
        }
      }
      event "TWS": Value Change {
        n195 = event-data() -> ("NewVal"=w440:bool)  [unwired: 6 out]
        n196 = case shown="True" w440 {
          tunnel: w443 -> [w444 w451]
          tunnel: w442 -> [_ w450]
          tunnel: [w444 w448] -> w441
          frame False {
          }
          frame True {
            n197 = for {
              tunnel: w451 -> [w467]
              tunnel: w450 -> [w457]
              tunnel: "Firing Wavepoints" -> [w465] mode=indexing
              tunnel: [w458] -> w447
              i -> [w466]
              n198 = Array Size(array=w465) -> (size(s)=w464:i32)
              n199 = Increment(x=w466) -> (x+1=w463:i32)
              n200 = Initialize Array(w463, w464) -> (w461:i32[])
              n201 = Initialize Array(1, w464) -> (w460:i32[])
              n202 = call "TWS.vi"("System no."=w457, "Wavepoint"=w465, "Trigger value"=w461, "Switch"=w460, "error in"=w467) -> ("error out"=w459:errorcluster)  [unwired: 14 out]
              n203 = call "Wait for controller ready.vi"("System no."=w457, "error in"=w459) -> ("error out"=w458:errorcluster)  [unwired: 2 in, 15 out]
            }
            n204 = local read "SubVI"() -> (w446:bool)
            n205 = case shown="False" w446 {
              tunnel: [w455 w456] -> w448
              tunnel: w447 -> [w452 w456]
              frame False {
                n206 = control-ref of="TWS?"() -> (w454:refnum<vi>)
                n207 = property class="Bool (strict)"(reference=w454, error in=w452, "Value (Signaling)"=TRUE ("TWC")) -> (error out=w455:errorcluster)  [unwired: 1 out]
              }
              frame True {
              }
            }
            n208 = local write "TWS"(FALSE ("TWS")) -> ()
          }
        }
      }
      event "TWC": Value Change {
        n209 = event-data() -> ("NewVal"=w468:bool)  [unwired: 6 out]
        n210 = case shown="True" w468 {
          tunnel: w471 -> [w472 w479]
          tunnel: [w472 w478] -> w470
          tunnel: w469 -> [_ w475]
          frame False {
          }
          frame True {
            n211 = call "TWC.vi"("System no."=w475, "error in"=w479) -> ("error out"=w477:errorcluster)  [unwired: 17 out]
            n212 = call "Wait for controller ready.vi"("System no."=w475, "error in"=w477) -> ("error out"=w476:errorcluster)  [unwired: 2 in, 15 out]
            n213 = local write "TWC"(FALSE ("TWC")) -> ()
            n214 = local read "SubVI"() -> (w474:bool)
            n215 = case shown="False" w474 {
              tunnel: [w481 w484] -> w478
              tunnel: w476 -> [w480 w484]
              frame False {
                n216 = control-ref of="TWS?"() -> (w483:refnum<vi>)
                n217 = property class="Bool (strict)"(reference=w483, error in=w480, "Value (Signaling)"=TRUE ("TWC")) -> (error out=w481:errorcluster)  [unwired: 1 out]
              }
              frame True {
              }
            }
          }
        }
      }
      event "Axis": Value Change {
        # "Not supported by this controller"
        n218 = event-data() -> ()  [unwired: 7 out]
        n219 = for {
          tunnel: "Axis" -> [w500] mode=indexing
          tunnel: w492 -> [w499]
          tunnel: [w496] -> w489 mode=indexing
          tunnel: [w495] -> w487 mode=indexing
          i -> [w498]
          n220 = Increment(x=w498) -> (x+1=w497:i32)
          n221 = Index Array(array=w499, index=w500) -> (element=w495:string)
          n222 = Number To Decimal String(number=w497) -> (decimal integer string=w496:string)  [unwired: 1 out]
        }
        n223 = Array Size(array="Axis") -> (size(s)=w494:i32)
        n224 = Initialize Array(T5."Axis", w494) -> (w490:T7)
        n225 = call "CTO.vi"("System no."=w488, "TriggerOut to set"=w489, "error in"=w485, "CTO parameter ID"=w490, "Parameter value"=w487) -> ("error out"=w486:errorcluster)  [unwired: 1 in, 13 out]
      }
      event "Write points": Value Change {
        n226 = event-data() -> ("NewVal"=w507:bool)  [unwired: 6 out]
        n227 = local read "Wavetable"() -> (w503:u16)
        n228 = case shown="True" w507 {
          tunnel: w506 -> [w508 w532]
          tunnel: [w508 w519] -> w502
          tunnel: w505 -> [_ w513]
          tunnel: w504 -> [_ w536]
          tunnel: w503 -> [_ w520]
          tunnel: w501 -> [_ w512]
          frame False {
          }
          frame True {
            w537 = u16 3 items=["SIN", "POL", "TAN", "PNT", "SIN_P", "LIN", "RAMP"] ("Waveform")
            w518 = TRUE ("All axes?")
            # "Generate ramp"
            n229 = call "TMN?.vi"("System no."=w513, "All axes?"=w518, "error in"=w532) -> ("Minimum travel limit"=w533:dbl[], "error out"=w530:errorcluster)  [unwired: 2 in, 13 out]
            n230 = Index Array(array=w533, index=w520) -> (element=w527:dbl)
            n231 = call "TMX?.vi"("System no."=w513, "All axes?"=w518, "error in"=w530) -> ("Maximum travel limit"=w531:dbl[], "error out"=w525:errorcluster)  [unwired: 2 in, 13 out]
            n232 = local read "N"() -> (w523:i32)
            n233 = local read "Segm.Length"() -> (w511:i32)
            n234 = local read "Append?"() -> (w522:bool)
            n235 = local read "Xo"() -> (w521:i32)
            n236 = local read "Add?"() -> (w517:bool)
            n237 = Index Array(array=w531, index=w520) -> (element=w529:dbl)
            n238 = Index Array(array=w536, index=w520) -> (element=w535:string)
            n239 = Subtract(x=w529, y=w527) -> (x-y=w528:dbl)
            n240 = Build Array(w535) -> (w534:string[])
            n241 = Divide(x=w528, y=w523) -> (x/y=w526:dbl)
            n242 = for {
              N: w523 -> [_]
              tunnel: w527 -> [w544]
              tunnel: w526 -> [w546]
              tunnel: [w543] -> w524 mode=indexing
              i -> [w547]
              n243 = Multiply(x=w547, y=w546) -> (x*y=w545:dbl)
              n244 = Add(x=w545, y=w544) -> (x+y=w543:dbl)
            }
            n245 = Bundle(w524) -> (w516:cluster{dbl[]})  [unwired: 1 in]
            "PNT parameters (indicator)" <- w516
            n246 = call "WAV.vi"("System no."=w513, "Waveform"=w537, "Affected axes"=w534, "Append? (&)"=w522, "Add? (+)"=w517, "error in"=w525, "Xo"=w521, "N"=w523, "Nmax for PNT"=w512, "Segment length"=w511, "PNT Parameters"=w516) -> ("error out"=w515:errorcluster)  [unwired: 7 in, 9 out]
            n247 = call "Wait for controller ready.vi"("System no."=w513, "error in"=w515) -> ("error out"=w514:errorcluster)  [unwired: 2 in, 15 out]
            n248 = local read "SubVI"() -> (w510:bool)
            n249 = case shown="False" w510 {
              tunnel: [w540 w542] -> w519
              tunnel: w514 -> [w538 w542]
              frame False {
                n250 = control-ref of="GWD?"() -> (w539:refnum<vi>)
                n251 = property class="Bool (strict)"(reference=w539, error in=w538, "Value (Signaling)"=TRUE ("GWD?")) -> (error out=w540:errorcluster)  [unwired: 1 out]
              }
              frame True {
              }
            }
            n252 = local write "Write points"(FALSE ("Write points")) -> ()
          }
        }
      }
      event "DDL enable": Value Change {
        w554 = 128
        n253 = event-data() -> ("NewVal"=w556:bool[])  [unwired: 6 out]
        n254 = Boolean To (0,1)(Boolean=w556) -> (0, 1=w555:i16[])
        n255 = local read "WGO mode"() -> (w553:i32[])
        n256 = Multiply(x=w555, y=w554) -> (x*y=w551:i32[])
        n257 = Not(x=w554) -> (.not. x?=w552:i32)
        n258 = And(x=w553, y=w552) -> (x .and. y?=w550:i32[])
        n259 = Or(x=w550, y=w551) -> (x .or. y?=w549:i32[])
        n260 = local write "WGO mode"(w549) -> ()
      }
      event "DDL init": Value Change {
        w562 = 64
        n261 = event-data() -> ("NewVal"=w560:bool[])  [unwired: 6 out]
        n262 = local read "WGO mode"() -> (w558:i32[])
        n263 = Boolean To (0,1)(Boolean=w560) -> (0, 1=w561:i16[])
        n264 = Multiply(x=w561, y=w562) -> (x*y=w564:i32[])
        n265 = Not(x=w562) -> (.not. x?=w563:i32)
        n266 = And(x=w558, y=w563) -> (x .and. y?=w565:i32[])
        n267 = Or(x=w565, y=w564) -> (x .or. y?=w559:i32[])
        n268 = local write "WGO mode"(w559) -> ()
      }
      event "Start at\nEndpoint": Value Change {
        w571 = 256
        n269 = event-data() -> ("NewVal"=w567:bool[])  [unwired: 6 out]
        n270 = local read "WGO mode"() -> (w568:i32[])
        n271 = Boolean To (0,1)(Boolean=w567) -> (0, 1=w570:i16[])
        n272 = Multiply(x=w570, y=w571) -> (x*y=w573:i32[])
        n273 = Not(x=w571) -> (.not. x?=w572:i32)
        n274 = And(x=w568, y=w572) -> (x .and. y?=w574:i32[])
        n275 = Or(x=w574, y=w573) -> (x .or. y?=w569:i32[])
        n276 = local write "WGO mode"(w569) -> ()
      }
    }
  }
  n277 = local read "SubVI"() -> (w16:bool)
  n278 = case shown="True" w16 {
    tunnel: [w575 w576] -> w36
    tunnel: "Programmatic events" -> [_ w577]
    tunnel: w14 -> [w575 _]
    frame False {
    }
    frame True {
      n279 = Build Array (concatenate)(w577, T8."Exit VI" ("Enum")) -> (w576:T1)
    }
  }
  n280 = Wait on Notification(notifier=w28, error in (no error)=w31) -> (notifier out=w29:refnum<notifier>, error out=w30:errorcluster)  [unwired: 4 out]
  n281 = for {
    tunnel: w36 -> [w582] mode=indexing
    tunnel: w29 -> [w581]
    shift-right: [w580] -> w26
    shift-left: w30 -> [w579]
    n282 = case shown="\"Write sine\"" w582 {
      tunnel: w581 -> [_ w587 w596 w603 w610 w616 w621 w629 w638 w642 w648 w657 w662 w671 w678 w684 w691 w699 w706 w711]
      tunnel: [w583 w588 w594 w601 w609 w613 w620 w631 w637 w644 w650 w658 w664 w670 w677 w685 w690 w700 w708 w714] -> w580
      tunnel: w579 -> [w583 w585 w595 w602 w608 w615 w622 w630 w636 w643 w651 w659 w665 w672 w679 w687 w694 w701 w707 w715]
      frame "Exit VI", Default {
        n283 = local write "Stop"(TRUE ("Stop")) -> ()
      }
      frame "Set trigger mode" {
        n284 = control-ref of="CTO"() -> (w586:refnum<vi>)
        n285 = property class="Bool (strict)"(reference=w586, error in=w585, "Value (Signaling)"=TRUE ("GWD?")) -> (error out=w590:errorcluster)  [unwired: 1 out]
        n286 = Wait on Notification(notifier=w587, ignore previous (F)=TRUE, error in (no error)=w590) -> (error out=w588:errorcluster)  [unwired: 4 out]
      }
      frame "Set recordtable rate" {
        n287 = local read "Recordtable rate"() -> (w593:i32)
        n288 = control-ref of="Recordtable rate"() -> (w592:refnum<vi>)
        n289 = property class="DigNum (strict)"(reference=w592, error in=w595, "Value (Signaling)"=w593) -> (error out=w598:errorcluster)  [unwired: 1 out]
        n290 = Wait on Notification(notifier=w596, ignore previous (F)=TRUE, error in (no error)=w598) -> (error out=w594:errorcluster)  [unwired: 4 out]
      }
      frame "Set wavetable rate" {
        n291 = local read "Wavetable rate"() -> (w600:i32[])
        n292 = control-ref of="Wavetable rate"() -> (w599:refnum<vi>)
        n293 = property class="Arr (strict)"(reference=w599, error in=w602, "Value (Signaling)"=w600) -> (error out=w605:errorcluster)  [unwired: 1 out]
        n294 = Wait on Notification(notifier=w603, ignore previous (F)=TRUE, error in (no error)=w605) -> (error out=w601:errorcluster)  [unwired: 4 out]
      }
      frame "Write sine" {
        n295 = control-ref of="Write sine"() -> (w607:refnum<vi>)
        n296 = property class="Bool (strict)"(reference=w607, error in=w608, "Value (Signaling)"=TRUE ("GWD?")) -> (error out=w611:errorcluster)  [unwired: 1 out]
        n297 = Wait on Notification(notifier=w610, ignore previous (F)=TRUE, error in (no error)=w611) -> (error out=w609:errorcluster)  [unwired: 4 out]
      }
      frame "Read wavetable" {
        n298 = control-ref of="GWD?"() -> (w614:refnum<vi>)
        n299 = property class="Bool (strict)"(reference=w614, error in=w615, "Value (Signaling)"=TRUE ("GWD?")) -> (error out=w618:errorcluster)  [unwired: 1 out]
        n300 = Wait on Notification(notifier=w616, ignore previous (F)=TRUE, error in (no error)=w618) -> (error out=w613:errorcluster)  [unwired: 4 out]
      }
      frame "Read recordtable" {
        n301 = control-ref of="DRR?"() -> (w623:refnum<vi>)
        n302 = property class="Bool (strict)"(reference=w623, error in=w622, "Value (Signaling)"=TRUE ("GWD?")) -> (error out=w625:errorcluster)  [unwired: 1 out]
        n303 = Wait on Notification(notifier=w621, ignore previous (F)=TRUE, error in (no error)=w625) -> (error out=w620:errorcluster)  [unwired: 4 out]
      }
      frame "Enable/disable wavegen" {
        n304 = control-ref of="Enabled"() -> (w628:refnum<vi>)
        n305 = local read "Enabled"() -> (w627:bool[])
        n306 = property class="Arr (strict)"(reference=w628, error in=w630, "Value (Signaling)"=w627) -> (error out=w633:errorcluster)  [unwired: 1 out]
        n307 = Wait on Notification(notifier=w629, ignore previous (F)=TRUE, error in (no error)=w633) -> (error out=w631:errorcluster)  [unwired: 4 out]
      }
      frame "Set number of wavegen cycles" {
        n308 = local read "# WG cycles"() -> (w634:i32[])
        n309 = control-ref of="# WG cycles"() -> (w635:refnum<vi>)
        n310 = property class="Arr (strict)"(reference=w635, error in=w636, "Value (Signaling)"=w634) -> (error out=w639:errorcluster)  [unwired: 1 out]
        n311 = Wait on Notification(notifier=w638, ignore previous (F)=TRUE, error in (no error)=w639) -> (error out=w637:errorcluster)  [unwired: 4 out]
      }
      frame "Clear wavetable" {
        n312 = control-ref of="WCL"() -> (w641:refnum<vi>)
        n313 = property class="Bool (strict)"(reference=w641, error in=w643, "Value (Signaling)"=TRUE ("GWD?")) -> (error out=w646:errorcluster)  [unwired: 1 out]
        n314 = Wait on Notification(notifier=w642, ignore previous (F)=TRUE, error in (no error)=w646) -> (error out=w644:errorcluster)  [unwired: 4 out]
      }
      frame "Configure data recorder" {
        n315 = control-ref of="DRC"() -> (w649:refnum<vi>)
        n316 = property class="Bool (strict)"(reference=w649, error in=w651, "Value (Signaling)"=TRUE ("GWD?")) -> (error out=w653:errorcluster)  [unwired: 1 out]
        n317 = Wait on Notification(notifier=w648, ignore previous (F)=TRUE, error in (no error)=w653) -> (error out=w650:errorcluster)  [unwired: 4 out]
      }
      frame "Assign wavetable to wavegen" {
        n318 = control-ref of="Wavegen"() -> (w656:refnum<vi>)
        n319 = local read "Wavegen"() -> (w655:i32[])
        n320 = property class="Arr (strict)"(reference=w656, error in=w659, "Value (Signaling)"=w655) -> (error out=w661:errorcluster)  [unwired: 1 out]
        n321 = Wait on Notification(notifier=w657, ignore previous (F)=TRUE, error in (no error)=w661) -> (error out=w658:errorcluster)  [unwired: 4 out]
      }
      frame "Read trigger points" {
        n322 = control-ref of="TWS?"() -> (w663:refnum<vi>)
        n323 = property class="Bool (strict)"(reference=w663, error in=w665, "Value (Signaling)"=TRUE ("GWD?")) -> (error out=w667:errorcluster)  [unwired: 1 out]
        n324 = Wait on Notification(notifier=w662, ignore previous (F)=TRUE, error in (no error)=w667) -> (error out=w664:errorcluster)  [unwired: 4 out]
      }
      frame "Set trigger points" {
        n325 = control-ref of="TWS"() -> (w669:refnum<vi>)
        n326 = property class="Bool (strict)"(reference=w669, error in=w672, "Value (Signaling)"=TRUE ("GWD?")) -> (error out=w674:errorcluster)  [unwired: 1 out]
        n327 = Wait on Notification(notifier=w671, ignore previous (F)=TRUE, error in (no error)=w674) -> (error out=w670:errorcluster)  [unwired: 4 out]
      }
      frame "Clear trigger points" {
        n328 = control-ref of="TWC"() -> (w676:refnum<vi>)
        n329 = property class="Bool (strict)"(reference=w676, error in=w679, "Value (Signaling)"=TRUE ("GWD?")) -> (error out=w681:errorcluster)  [unwired: 1 out]
        n330 = Wait on Notification(notifier=w678, ignore previous (F)=TRUE, error in (no error)=w681) -> (error out=w677:errorcluster)  [unwired: 4 out]
      }
      frame "Assign axes to triggerlines" {
        n331 = local read "Axis"() -> (w683:u16[])
        n332 = control-ref of="Axis"() -> (w686:refnum<vi>)
        n333 = property class="Arr (strict)"(reference=w686, error in=w687, "Value (Signaling)"=w683) -> (error out=w689:errorcluster)  [unwired: 1 out]
        n334 = Wait on Notification(notifier=w684, ignore previous (F)=TRUE, error in (no error)=w689) -> (error out=w685:errorcluster)  [unwired: 4 out]
      }
      frame "Write ramp waveform" {
        n335 = control-ref of="Write points"() -> (w693:refnum<vi>)
        n336 = property class="Bool (strict)"(reference=w693, error in=w694, "Value (Signaling)"=TRUE ("GWD?")) -> (error out=w696:errorcluster)  [unwired: 1 out]
        n337 = Wait on Notification(notifier=w691, ignore previous (F)=TRUE, error in (no error)=w696) -> (error out=w690:errorcluster)  [unwired: 4 out]
      }
      frame "Set DDL enable" {
        n338 = local read "DDL enable"() -> (w697:bool[])
        n339 = control-ref of="DDL enable"() -> (w698:refnum<vi>)
        n340 = property class="Arr (strict)"(reference=w698, error in=w701, "Value (Signaling)"=w697) -> (error out=w703:errorcluster)  [unwired: 1 out]
        n341 = Wait on Notification(notifier=w699, ignore previous (F)=TRUE, error in (no error)=w703) -> (error out=w700:errorcluster)  [unwired: 4 out]
      }
      frame "Set DDL init" {
        n342 = control-ref of="DDL init"() -> (w705:refnum<vi>)
        n343 = local read "DDL init"() -> (w704:bool[])
        n344 = property class="Arr (strict)"(reference=w705, error in=w707, "Value (Signaling)"=w704) -> (error out=w710:errorcluster)  [unwired: 1 out]
        n345 = Wait on Notification(notifier=w706, ignore previous (F)=TRUE, error in (no error)=w710) -> (error out=w708:errorcluster)  [unwired: 4 out]
      }
      frame "Set Start at endpoint" {
        n346 = local read "Start at\nEndpoint"() -> (w712:bool[])
        n347 = control-ref of="Start at\nEndpoint"() -> (w713:refnum<vi>)
        n348 = property class="Arr (strict)"(reference=w713, error in=w715, "Value (Signaling)"=w712) -> (error out=w717:errorcluster)  [unwired: 1 out]
        n349 = Wait on Notification(notifier=w711, ignore previous (F)=TRUE, error in (no error)=w717) -> (error out=w714:errorcluster)  [unwired: 4 out]
      }
    }
  }
  n350 = local read "SubVI"() -> (w5:bool)
  n351 = for {
    tunnel: [0] -> w43 mode=indexing
    tunnel: w42 -> [_] mode=indexing
  }
  n352 = local write "Stop"(w35) -> ()
  n353 = Release Notifier(notifier=w32) -> ()  [unwired: 1 in, 4 out]
  n354 = call "CTO.vi"("System no."=w19, "TriggerOut to set"=w37, "error in"=w41, "CTO parameter ID"=w38, "Parameter value"=w39) -> ("error out"=w40:errorcluster)  [unwired: 1 in, 13 out]
  n355 = case shown="False" w5 {
    tunnel: [w723 w724] -> w54
    tunnel: w43 -> [w722 _]
    tunnel: w42 -> [w721 _]
    tunnel: w40 -> [w720 w724]
    tunnel: w19 -> [w719 _]
    frame False {
      n356 = call "WGO.vi"("System no."=w719, "Affected axes"=w721, "WGO Parameter"=w722, "error in"=w720) -> ("error out"=w723:errorcluster)  [unwired: 6 in, 9 out]
    }
    frame True {
    }
  }
  n357 = call "ERR?.vi"("System no."=w19, "error in"=w54) -> ("error out"=w55:errorcluster)  [unwired: 17 out]
  n358 = call "GCSTranslateError.vi"("error in"=w55) -> ("error out"=w27:errorcluster)  [unwired: 18 out]
  n359 = Merge Errors(w27, w26) -> (w25:errorcluster)
  n360 = local write "Error out"(w25) -> ()
